vi "Cross Power (DBL).vi"(2 "Y":dbl[](array[numeric]), 3 "X":dbl[](array[numeric])) -> (0 "error":i32, 1 "Sxy":cdb[](array[numeric]))   [LabVIEW 2010, in "NI_AALPro.lvlib"]
doc: "Computes the cross power spectrum, <B>Sxy</B>, of the input signals <B>X</B> and <B>Y</B>. Wire data to the <B>X</B> input to determine the polymorphic instance to use or manually select the instance."
uses:
  NI_AALPro.lvlib
  lvanlys.dll
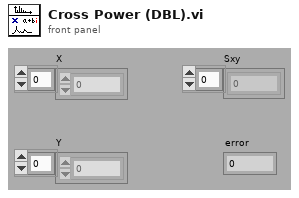
[diagram p1: front panel]
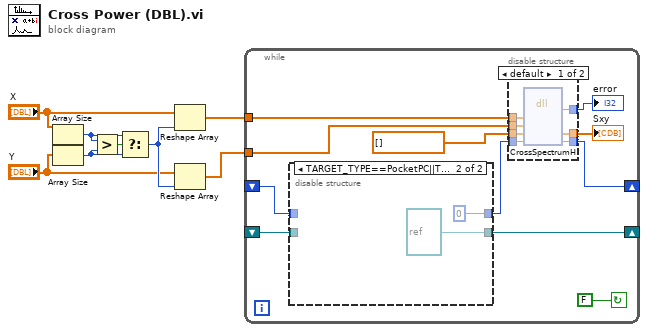
[diagram p0: block diagram]
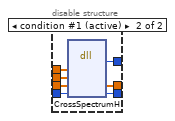
[diagram p2: hidden frame]
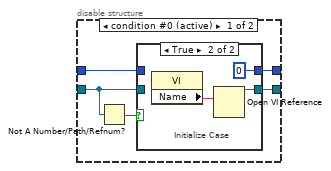
[diagram p3: hidden frame]
diagram:
  n1 = Array Size(array="X") -> (size(s)=w6:i32)
  n2 = Array Size(array="Y") -> (size(s)=w5:i32)
  n3 = Greater?(x=w6, y=w5) -> (0:w7:bool)
  n4 = Select(t=w6, s=w7, f=w5) -> (s? t:f=w8:i32)
  n5 = Reshape Array("X", w8) -> (w1:dbl[])
  n6 = Reshape Array("Y", w8) -> (w2:dbl[])
  n7 = while {
    tunnel: w2 -> [w16]
    shift-left: _ -> [w13]
    shift-right: [w15] -> _
    tunnel: w1 -> [w19]
    shift-right: [w11] -> _
    shift-left: _ -> [w12]
    stop <- FALSE continue-if-true
    n8 = disable-structure shown="TARGET_TYPE==PocketPC||TARGET_TYPE==PalmOS||TARGET_TYPE==FPGA||TARGET_TYPE==Embedded" {
      disable-tunnel: w12 -> [w36 _]
      disable-tunnel: [w37 refnum<vi> refnum ("VI Refnum")] -> w11
      disable-tunnel: w13 -> [w35 _]
      disable-tunnel: [w34 0 ("t")] -> w14
      frame condition #0 (active) {
        n9 = Not A Number/Path/Refnum?(number/path/refnum=w36) -> (NaN/Path/Refnum?=w38:bool)
        n10 = case shown="True" w38 {
          tunnel: [w40 w42] -> w37
          tunnel: w36 -> [w40 _]
          tunnel: w35 -> [w39 _]
          tunnel: [w39 0 ("error")] -> w34
          frame False {
          }
          frame True {
            # "Initialize Case"
            n11 = property class="VI"() -> ("Name"=w41:string)  [unwired: 2 in, 2 out]
            n12 = Open VI Reference(vi path=w41) -> (vi reference=w42:refnum<vi>)  [unwired: 5 in, 1 out]
          }
        }
      }
      frame condition #1 {
      }
    }
    n13 = disable-structure shown="default" {
      disable-tunnel: w19 -> [w26 w33]
      disable-tunnel: [w25 w32] -> w18
      disable-tunnel: [w24 w31] -> w10
      disable-tunnel: w16 -> [w23 w30]
      disable-tunnel: [w22 w29] -> w15
      disable-tunnel: w14 -> [w21 w28]
      disable-tunnel: cdb[] [] ("Sxy") -> [w20 w27]
      frame condition #0 {
        n14 = dll-call lib="C:/Program Files/National Instruments/LabVIEW 2010/resource/lvanlys.dll" fn="CrossSpectrumH"("X"=w26, "Y"=w23, w20, "tbl"=w21) -> (w25:i32, w24:cdb[], "tbl"=w22:i32)  [unwired: 5 in, 2 out]
      }
      frame condition #1 (active) {
        n15 = dll-call lib="C:/Program Files/National Instruments/LabVIEW 2010/resource/lvanlys.dll" fn="CrossSpectrumH"("xH"=w33, "yH"=w30, "zH"=w27, "tbl"=w28) -> ("return type"=w32:i32, "zH"=w31:cdb[], "tbl"=w29:i64)  [unwired: 5 in, 2 out]
      }
    }
    "Sxy" <- w10
    "error" <- w18
  }
